vi "S8300E_Chk_MCU_Version_WIH.vi"() -> ()   [LabVIEW 2011]
panel:
  out "FinalLOG2":string
  out "Final-log-1":string
  out "temp-log-1":string
  out "FinalLOG1":string
  out "LOG1":string
  out "log2":string
  out "begin MCU_ID time":u32
  out "Begin FW chk time":u32
  out "log-1":string
  out "cmd-list":T1(array[cluster])
  out "MCU_DEV_ID":string
  out "MCU_FW_VER":string
  out "Debug View":string
  out "MSG List":string[](array[string])
  out "VISA resource name out":refnum<visa-resource-name>
  out "BEGIN TIME":u32
  out "進行狀況":string
  # "Error Code:MCU_FW\nError Code:MCU_ID"
  # "2015-5-28"
  # "S8300E Check MCU Version"
  # "COM9 :Baud-Rate:115200"
  # "Step1:Check PIC MCU Firmware Version\nStep2:Check PIC MCU Device ID"
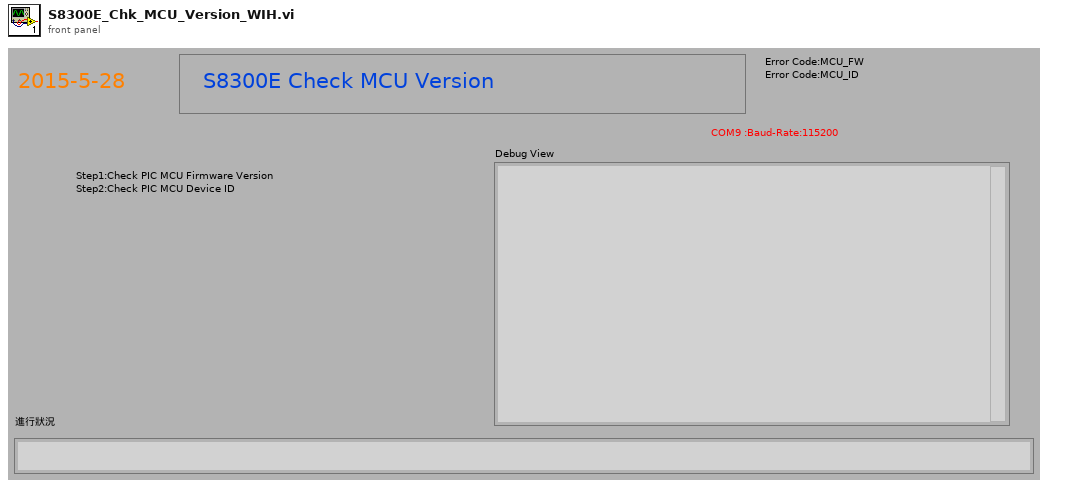
[diagram p1: front panel]
types:
  T1 = cluster{string, string, "MCU_DEV_ID":string, string}[]
  T2 = cluster{string, string, "MCU_FW_VER":string, string}
  T3 = cluster{string, string, "MCU_DEV_ID":string, string}
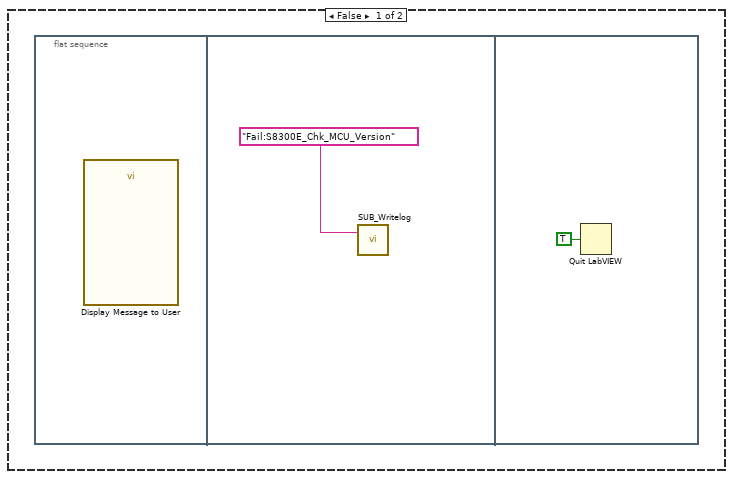
[diagram p2: hidden frame]
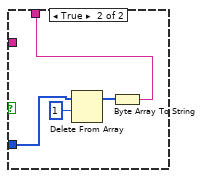
[diagram p3: hidden frame]
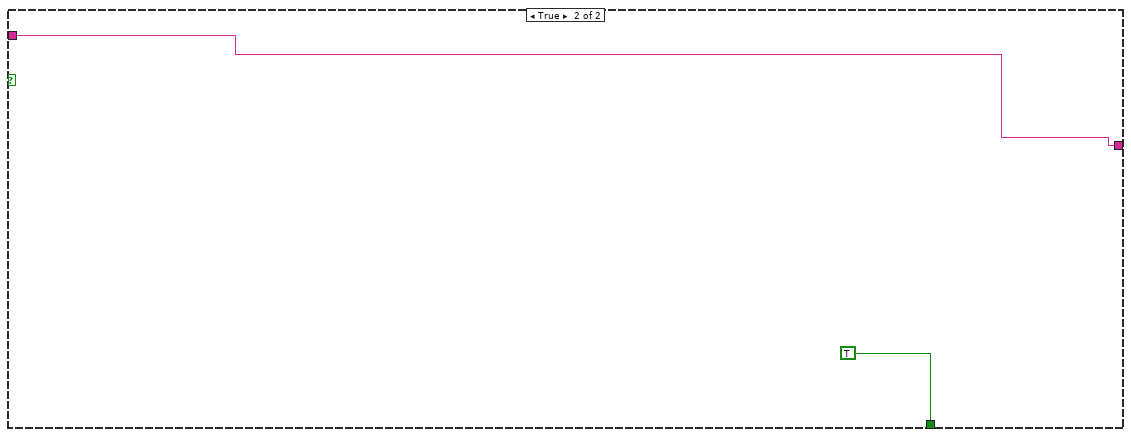
[diagram p6: hidden frame]
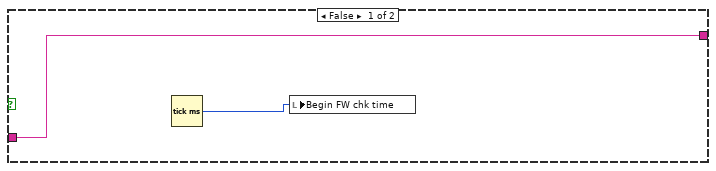
[diagram p7: hidden frame]
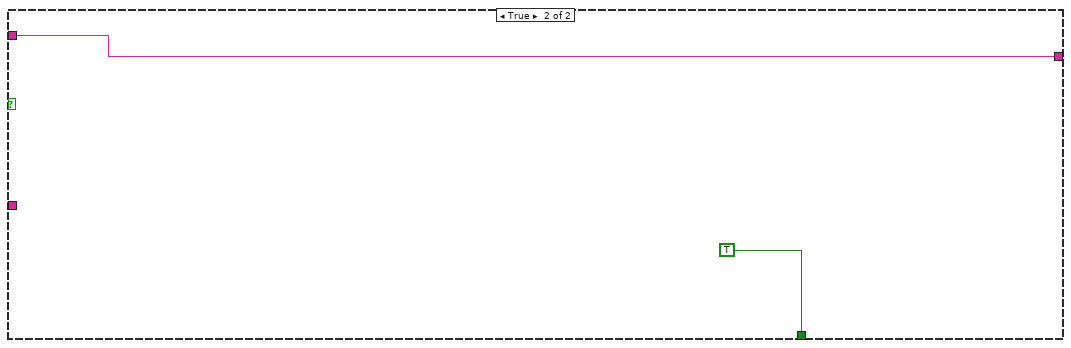
[diagram p8: hidden frame]
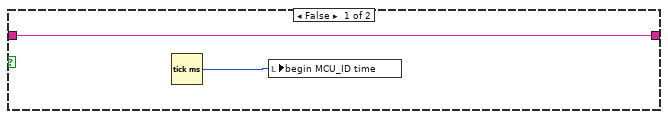
[diagram p9: hidden frame]
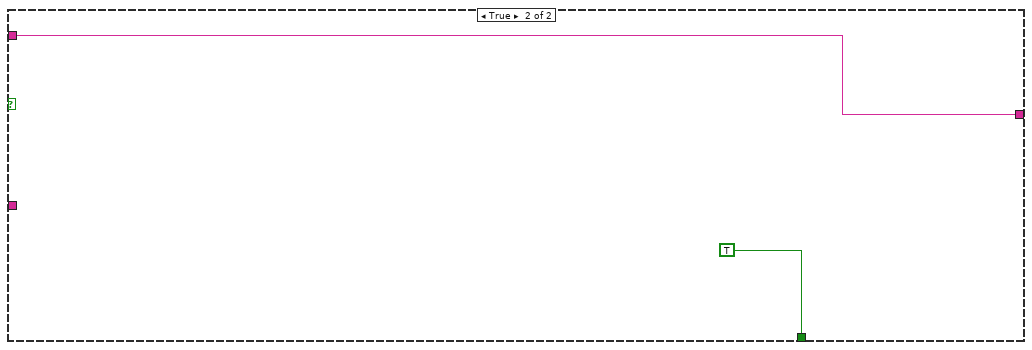
[diagram p10: hidden frame]
diagram:
  n1 = flat-sequence {
    tunnel: [w48] -> w1
    tunnel: w1 -> [w49]
    frame #0 {
      n2 = Tick Count (ms)() -> (millisecond timer value=→"BEGIN TIME":u32)
    }
    frame #1 {
      n3 = Request Deallocation(TRUE ("flag")) -> ()
      n4 = property on="進行狀況" class="Str"("Blinking"=TRUE) -> ()  [unwired: 2 in, 2 out]
      "進行狀況" <- "進入測試準備中...." ("進行狀況")
      "Debug View" <- ""
    }
    frame #2 {
      n5 = call "SUB_SearchFile_inFolder.vi"("Search Filename in Folder"="S8300E_sfcs_misc.txt") -> ("File Existing True/Flase"=w7:bool)  [unwired: 1 in]
      n6 = case shown="True" w7 {
        frame False {
          n7 = flat-sequence {
            frame #0 {
              n8 = call "Display Message to User"() -> ()  [unwired: 10 in, 2 out]
            }
            frame #1 {
              n9 = call "SUB_Writelog.vi"("Pass/Fail"="Fail:S8300E_Chk_MCU_Version") -> ()  [unwired: 2 in]
            }
            frame #2 {
              n10 = Quit LabVIEW(quit? (T)=TRUE) -> ()
            }
          }
        }
        frame True {
          n11 = call "SUB_Read_specifFile.vi"("name or relative path"="S8300E_sfcs_misc.txt" ("Search Filename in Folder")) -> ("text"=w21:string)  [unwired: 1 in, 1 out]
          n12 = call "SUB_FindSpecificString.vi"("Find this String"="UUT_MCU_FW_VERSION=", "String data"=w21) -> ("before \"; \" string"=→"MCU_FW_VER":string, "Found"=w19:bool)  [unwired: 2 in]
          n13 = call "SUB_FindSpecificString.vi"("Find this String"="UUT_MCU_DEVICE_ID=", "String data"=w21) -> ("before \"; \" string"=w12:string, "Found"=w18:bool)  [unwired: 2 in]
          n14 = String To Byte Array(string=w12) -> (unsigned byte array=w13:u8[])
          n15 = Array Size(array=w13) -> (size(s)=w16:i32)
          n16 = Greater Or Equal?(x=w16, y=6) -> (x >= y?=w14:bool)
          n17 = case shown="False" w14 {
            tunnel: w13 -> [_ w28]
            tunnel: [w25 w26] -> w11
            tunnel: w12 -> [w25 _]
            frame False {
            }
            frame True {
              n18 = Delete From Array(array=w28, length=1) -> (array with subset deleted=w27:u8[])  [unwired: 1 in, 1 out]
              n19 = Byte Array To String(unsigned byte array=w27) -> (string=w26:string)
            }
          }
          "MCU_DEV_ID" <- w11
          n20 = And(x=w19, y=w18) -> (x .and. y?=w17:bool)
          n21 = case shown="False" w17 {
            frame False {
              n22 = flat-sequence {
                frame #0 {
                  n23 = call "Display Message to User2"() -> ()  [unwired: 10 in, 2 out]
                }
                frame #1 {
                  n24 = call "SUB_Writelog.vi"("Pass/Fail"="Fail:S8300E_Chk_MCU_Version") -> ()  [unwired: 2 in]
                }
                frame #2 {
                  n25 = Quit LabVIEW(quit? (T)=TRUE) -> ()
                }
              }
            }
            frame True {
            }
          }
        }
      }
    }
    frame #3 {
      n26 = local read "MCU_FW_VER"() -> (w39:string)
      n27 = local read "MCU_DEV_ID"() -> (w36:string)
      n28 = Bundle("./ver.sh -m", "PASSED=", "MCU_FW_VER"=w39, "MCU_FW") -> (w42:T2)  [unwired: 1 in]
      n29 = Bundle("./ver.sh -d", "PASSED=", "MCU_DEV_ID"=w36, "MCU_ID") -> (w35:T3)  [unwired: 1 in]
      n30 = Build Array(w42, w35) -> (→"cmd-list":T1)
      n31 = Build Array("正在處理 Buttun 初始值") -> (→"MSG List":string[])
    }
    frame #4 {
      n32 = call "SUB_COM1_CLOSE.vi"("VISA resource name"=refnum<visa-resource-name> "COM9") -> ()  [unwired: 3 in]
    }
    frame #5 {
      n33 = call "SUB_COM9_INIT.vi"("baud rate"=u32 115200) -> ("VISA resource name out"=→"VISA resource name out":refnum<visa-resource-name>)  [unwired: 1 in, 1 out]
    }
    frame #6 {
      n34 = Tick Count (ms)() -> (millisecond timer value=w48:u32)
    }
    frame #7 {
      n35 = while {
        shift-right: [w59] -> _
        shift-left: "" -> [w60]
        tunnel: w49 -> [w54]
        stop <- w57 stop-if-true
        n36 = local read "VISA resource name out"() -> (w64:refnum<visa-resource-name>)
        n37 = call "SUB_COM1Wrt.vi"("VISA resource name"=w64, "write buffer"="\r") -> ("duplicate VISA resource name"=w63:refnum<visa-resource-name>)  [unwired: 1 in, 1 out]
        n38 = Tick Count (ms)() -> (millisecond timer value=w55:u32)
        n39 = Subtract(x=w55, y=w54) -> (x-y=w53:u32)
        n40 = Greater Or Equal?(x=w53, y=u32 5000) -> (x >= y?=w51:bool)
        n41 = call "SUB_ContinueCom1Read.vi"("Numeric"=1200, "duplicate VISA resource name 2"=w63) -> ("String"=w61:string)  [unwired: 1 in, 2 out]
        n42 = Concatenate Strings(w60, w61) -> (w59:string)
        n43 = call "SUB_FindSpecificString.vi"("Find this String"="S8300E", "String data"=w59) -> ("Found"=w56:bool)  [unwired: 2 in, 1 out]
        n44 = Or(x=w56, y=w51) -> (x .or. y?=w57:bool)
      }
    }
    frame #8 {
      n45 = while {
        shift-right: [w71] -> w66
        shift-left: "" -> [w70]
        stop <- w75 stop-if-true
        w72 = "S8300E" ("Find this String")
        n46 = local read "VISA resource name out"() -> (w68:refnum<visa-resource-name>)
        n47 = call "SUB_COM1Wrt.vi"("VISA resource name"=w68, "write buffer"="\r") -> ("duplicate VISA resource name"=w78:refnum<visa-resource-name>)  [unwired: 1 in, 1 out]
        n48 = Tick Count (ms)() -> (millisecond timer value=w77:u32)
        n49 = call "SUB_READ_COM1_FindString_timeout.vi"("Find this String"=w72, "Timeout Seccond"=3.0, "Begin time"=w77, "duplicate VISA resource name 2"=w78) -> ("Output String"=w73:string)  [unwired: 1 in, 2 out]
        n50 = call "SUB_FindSpecificString.vi"("Find this String"=w72, "String data"=w73) -> ("Found"=w74:bool)  [unwired: 2 in, 1 out]
        n51 = case shown="False" w74 {
          tunnel: [w84 TRUE] -> w75
          tunnel: w73 -> [w82 w102]
          tunnel: [w80 w102] -> w69
          frame False {
            w83 = "UART無正確反應!需有S8300E字串" ("Status")
            n52 = Concatenate Strings(w83, w82) -> (w81:string)
            n53 = call "SUB_YESNO.vi"("Debug View"=w82, "Status"=w83) -> ("yes/no"=w87:enum32{"No Selection", "Yes", "No", "None"})  [unwired: 1 in]
            n54 = Equal?(x=w87, y=enum32{"No Selection", "Yes", "No", "None"}."No") -> (x = y?=w85:bool)
            n55 = case shown="True" w85 {
              tunnel: [_ w92] -> w84
              tunnel: w81 -> [w88 w91]
              tunnel: [w88 w90] -> w80
              frame False {
              }
              frame True {
                n56 = flat-sequence {
                  tunnel: w91 -> [w96]
                  tunnel: [w95] -> w89
                  tunnel: [w98] -> w90
                  tunnel: w89 -> [w98]
                  tunnel: [w101] -> w92
                  frame #0 {
                    w94 = "\n"
                    n57 = local read "LOG1"() -> (w93:string)
                    n58 = Concatenate Strings("Fail:S8300E_Chk_MCU_Version" ("Pass/Fail"), w94, w96, w94, w93) -> (w95:string)
                    n59 = call "SUB_Writelog.vi"("Pass/Fail"=w95) -> ()  [unwired: 2 in]
                  }
                  frame #1 {
                    n60 = call "SUB_SFCS_SendResult.vi"("ErrorCode"="UART", "PASS_Fail (1/0)"=i8 0) -> ()  [unwired: 1 out]
                  }
                  frame #2 {
                    w101 = TRUE ("quit? (T)")
                    n61 = Quit LabVIEW(quit? (T)=w101) -> ()
                  }
                }
              }
            }
          }
          frame True {
          }
        }
        n62 = Concatenate Strings(w70, w69) -> (w71:string)
        "LOG1" <- w71
      }
      "FinalLOG1" <- w66
    }
    frame #9 {
      n63 = Tick Count (ms)() -> (millisecond timer value=→"Begin FW chk time":u32)
      n64 = local write "進行狀況"("Check MCU_FW...." ("進行狀況")) -> ()
    }
    frame #10 {
      n65 = while {
        shift-right: [w111] -> w106
        shift-left: "" -> [w110]
        stop <- w112 stop-if-true
        n66 = flat-sequence {
          tunnel: [w117] -> w114
          tunnel: [w116] -> w113
          tunnel: [w115] -> w108
          tunnel: w114 -> [w143]
          tunnel: w113 -> [w142]
          tunnel: [w141] -> w112
          tunnel: [w140] -> w109
          tunnel: w108 -> [w139]
          frame #0 {
            n67 = while {
              shift-right: [w120] -> w115
              shift-left: "" -> [w134]
              tunnel: [w127] -> w117
              tunnel: [w126] -> w116
              stop <- w132 stop-if-true
              n68 = local read "VISA resource name out"() -> (w119:refnum<visa-resource-name>)
              n69 = local read "Begin FW chk time"() -> (w125:u32)
              n70 = local read "MCU_FW_VER"() -> (w124:string)
              n71 = Concatenate Strings("./ver.sh -m", "\r") -> (w123:string)
              n72 = call "SUB_COM1Wrt.vi"("VISA resource name"=w119, "write buffer"=w123) -> ("duplicate VISA resource name"=w136:refnum<visa-resource-name>)  [unwired: 1 in, 1 out]
              n73 = Tick Count (ms)() -> (millisecond timer value=w131:u32)
              n74 = call "SUB_ContinueCom1Read.vi"("Numeric"=9600, "duplicate VISA resource name 2"=w136) -> ("String"=w122:string)  [unwired: 1 in, 2 out]
              n75 = Concatenate Strings("PASSED=", w124) -> (w126:string)
              n76 = Subtract(x=w131, y=w125) -> (x-y=w130:u32)
              n77 = Concatenate Strings(w123, w122) -> (w121:string)
              n78 = Concatenate Strings(w134, w121) -> (w120:string)
              "log-1" <- w120
              n79 = Greater Or Equal?(x=w130, y=u32 3000) -> (x >= y?=w128:bool)
              n80 = call "SUB_FindSpecificString.vi"("Find this String"=w126, "String data"=w120) -> ("Found"=w127:bool)  [unwired: 2 in, 1 out]
              n81 = Or(x=w127, y=w128) -> (x .or. y?=w132:bool)
            }
          }
          frame #1 {
            n82 = case shown="False" w143 {
              tunnel: w142 -> [w152 _]
              tunnel: [_ TRUE] -> w141
              tunnel: [w144 w165] -> w140
              tunnel: w139 -> [w148 w165]
              frame False {
                n83 = local read "log-1"() -> (w146:string)
                n84 = Concatenate Strings("系統須回" ("string"), w152) -> (w147:string)
                n85 = call "SUB_YESNO.vi"("Debug View"=w146, "Status"=w147) -> ("yes/no"=w150:enum32{"No Selection", "Yes", "No", "None"})  [unwired: 1 in]
                n86 = Equal?(x=w150, y=enum32{"No Selection", "Yes", "No", "None"}."No") -> (x = y?=w149:bool)
                n87 = Concatenate Strings(w148, w147, w146) -> (w145:string)
                n88 = case shown="True" w149 {
                  tunnel: w145 -> [w154 w156]
                  tunnel: [w154 _] -> w144
                  frame False {
                    n89 = Tick Count (ms)() -> (millisecond timer value=w155:u32)
                    n90 = local write "Begin FW chk time"(w155) -> ()
                  }
                  frame True {
                    n91 = flat-sequence {
                      tunnel: w156 -> [w158]
                      tunnel: [w164] -> _
                      frame #0 {
                        w159 = "\n"
                        n92 = local read "temp-log-1"() -> (w160:string)
                        n93 = Concatenate Strings("Fail:S8300E_Chk_MCU_Version" ("Pass/Fail"), w159, w160, w159, w158) -> (w157:string)
                        n94 = call "SUB_Writelog.vi"("Pass/Fail"=w157) -> ()  [unwired: 2 in]
                      }
                      frame #1 {
                        n95 = call "SUB_SFCS_SendResult.vi"("ErrorCode"="MCU_FW", "PASS_Fail (1/0)"=i8 0) -> ()  [unwired: 1 out]
                      }
                      frame #2 {
                        w164 = TRUE ("quit? (T)")
                        n96 = Quit LabVIEW(quit? (T)=w164) -> ()
                      }
                    }
                  }
                }
              }
              frame True {
              }
            }
          }
        }
        n97 = Concatenate Strings(w110, w109) -> (w111:string)
        "temp-log-1" <- w111
      }
      "Final-log-1" <- w106
    }
    frame #11 {
      n98 = Tick Count (ms)() -> (millisecond timer value=→"begin MCU_ID time":u32)
      n99 = local write "進行狀況"("Check MCU_ID...") -> ()
    }
    frame #12 {
      n100 = while {
        shift-right: [w174] -> w169
        shift-left: "" -> [w173]
        stop <- w175 stop-if-true
        n101 = flat-sequence {
          tunnel: [w180] -> w177
          tunnel: [w179] -> w176
          tunnel: [w178] -> w171
          tunnel: w177 -> [w206]
          tunnel: w176 -> [w205]
          tunnel: [w204] -> w175
          tunnel: [w203] -> w172
          tunnel: w171 -> [w202]
          frame #0 {
            n102 = while {
              shift-right: [w182] -> w178
              shift-left: "" -> [w197]
              tunnel: [w190] -> w180
              tunnel: [w189] -> w179
              stop <- w195 stop-if-true
              n103 = local read "VISA resource name out"() -> (w183:refnum<visa-resource-name>)
              n104 = local read "begin MCU_ID time"() -> (w188:u32)
              n105 = Concatenate Strings("./ver.sh -d", "\r") -> (w186:string)
              n106 = local read "MCU_DEV_ID"() -> (w187:string)
              n107 = call "SUB_COM1Wrt.vi"("VISA resource name"=w183, "write buffer"=w186) -> ("duplicate VISA resource name"=w199:refnum<visa-resource-name>)  [unwired: 1 in, 1 out]
              n108 = Tick Count (ms)() -> (millisecond timer value=w194:u32)
              n109 = call "SUB_ContinueCom1Read.vi"("Numeric"=9600, "duplicate VISA resource name 2"=w199) -> ("String"=w185:string)  [unwired: 1 in, 2 out]
              n110 = Concatenate Strings("PASSED=", w187) -> (w189:string)
              n111 = Subtract(x=w194, y=w188) -> (x-y=w193:u32)
              n112 = Concatenate Strings(w186, w185) -> (w184:string)
              n113 = Concatenate Strings(w197, w184) -> (w182:string)
              "log2" <- w182
              n114 = Greater Or Equal?(x=w193, y=u32 2000) -> (x >= y?=w191:bool)
              n115 = call "SUB_FindSpecificString.vi"("Find this String"=w189, "String data"=w182) -> ("Found"=w190:bool)  [unwired: 2 in, 1 out]
              n116 = Or(x=w190, y=w191) -> (x .or. y?=w195:bool)
            }
          }
          frame #1 {
            n117 = case shown="False" w206 {
              tunnel: w205 -> [w215 _]
              tunnel: [_ TRUE] -> w204
              tunnel: [w207 w227] -> w203
              tunnel: w202 -> [w211 w227]
              frame False {
                n118 = local read "log2"() -> (w209:string)
                n119 = Concatenate Strings("系統須回" ("string"), w215) -> (w210:string)
                n120 = call "SUB_YESNO.vi"("Debug View"=w209, "Status"=w210) -> ("yes/no"=w213:enum32{"No Selection", "Yes", "No", "None"})  [unwired: 1 in]
                n121 = Concatenate Strings(w211, w210, w209) -> (w208:string)
                n122 = Equal?(x=w213, y=enum32{"No Selection", "Yes", "No", "None"}."No") -> (x = y?=w212:bool)
                n123 = case shown="True" w212 {
                  tunnel: w208 -> [w217 w219]
                  tunnel: [w217 _] -> w207
                  frame False {
                    n124 = Tick Count (ms)() -> (millisecond timer value=w218:u32)
                    n125 = local write "begin MCU_ID time"(w218) -> ()
                  }
                  frame True {
                    n126 = flat-sequence {
                      tunnel: w219 -> [w221]
                      tunnel: [w226] -> _
                      frame #0 {
                        n127 = Concatenate Strings("Fail:S8300E_Chk_MCU_Version" ("Pass/Fail"), "\n", w221) -> (w220:string)
                        n128 = call "SUB_Writelog.vi"("Pass/Fail"=w220) -> ()  [unwired: 2 in]
                      }
                      frame #1 {
                        n129 = call "SUB_SFCS_SendResult.vi"("ErrorCode"="MCU_ID", "PASS_Fail (1/0)"=i8 0) -> ()  [unwired: 1 out]
                      }
                      frame #2 {
                        w226 = TRUE ("quit? (T)")
                        n130 = Quit LabVIEW(quit? (T)=w226) -> ()
                      }
                    }
                  }
                }
              }
              frame True {
              }
            }
          }
        }
        n131 = Concatenate Strings(w173, w172) -> (w174:string)
      }
      "FinalLOG2" <- w169
    }
    frame #13 {
      n132 = Request Deallocation(TRUE ("flag")) -> ()
    }
    frame #14 {
      n133 = call "SUB_COM1_CLOSE.vi"("VISA resource name"=refnum<visa-resource-name> "COM9") -> ()  [unwired: 3 in]
    }
    frame #15 {
      w233 = "***Not Good ***" ("replace string (\"\")")
      w241 = "\n"
      w245 = "\n"
      n134 = local read "FinalLOG2"() -> (w242:string)
      n135 = local read "BEGIN TIME"() -> (w247:u32)
      n136 = local read "Final-log-1"() -> (w243:string)
      n137 = Tick Count (ms)() -> (millisecond timer value=w246:u32)
      n138 = local read "FinalLOG1"() -> (w237:string)
      n139 = call "SUB_CAL_TESTTIME.vi"("Test Item name"="S8300E_Chk_MCU_Version", "Stop tick time"=w246, "Start tick time"=w247) -> ("Test Time output"=w244:string)  [unwired: 2 in]
      n140 = Concatenate Strings(w243, w241, w242, w241) -> (w240:string)
      n141 = Concatenate Strings("Pass:S8300E_Chk_MCU_Version", "\n", w237, w245, w240, w245, w245, w244) -> (w232:string)
      n142 = call "SUB_SEARCH_REPLACE_STR.vi"("replace string (\"\")"=w233, "search string"="FAILED", "input string"=w232) -> ("result string"=w235:string)  [unwired: 2 in]
      n143 = call "SUB_SEARCH_REPLACE_STR.vi"("replace string (\"\")"=w233, "search string"="FAIL", "input string"=w235) -> ("result string"=w231:string)  [unwired: 2 in]
      n144 = call "SUB_Writelog.vi"("Pass/Fail"=w231) -> ()  [unwired: 2 in]
    }
    frame #16 {
      n145 = Quit LabVIEW(quit? (T)=TRUE ("stop? (T)")) -> ()
    }
  }
